vi "TestPFGVName.vi"() -> (0 "error out":errorcluster, 2 "Pass":bool)   [LabVIEW 2015]
uses:
  TypeDef/RoomsActionEnum.ctl
  TypeDef/PersonnelActions.ctl
  LVClasses/Flags/Flags.lvclass
  LVClasses/Room/Room.lvclass
panel:
  out "Read Name":string
  out "Write Name":string
  out "Read Personnel":string
  out "Read Personnel 2":string
  in  "PUID":string="d1"
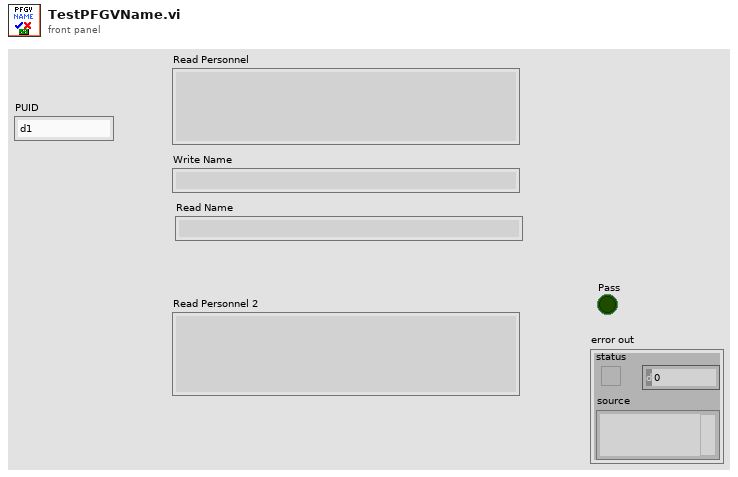
[diagram p1: front panel]
types:
  T1 = typedef "PersonnelActions.ctl" = enum16{"Init", "Read Personnel", "Add Personnel", "Remove Personnel", "Read Name", "Write Name", "Read Role", "Write Role", "Read PUID", "Write PUID", "Read Requests", "Add Requests", "Remove Requests"}
  T2 = typedef "RoomsActionEnum.ctl" = enum16{"Init", "Add Room", "Remove Room", "Read Room", "Read Flag", "Read Flag State", "Write Flag State", "Read Flag Color", "Write Flag Color", "Read Bed Vacant", "Write Bed Vacant", "Read Personnel", "Add Personnel", "Remove Personnel", "Read Requests", "Add Request", "Remove Request", "Read Beacon ID", "Write Beacon ID", "Write Bed URL", "Read Bed URL", "Read Rooms Numbers", "Write Flag"}
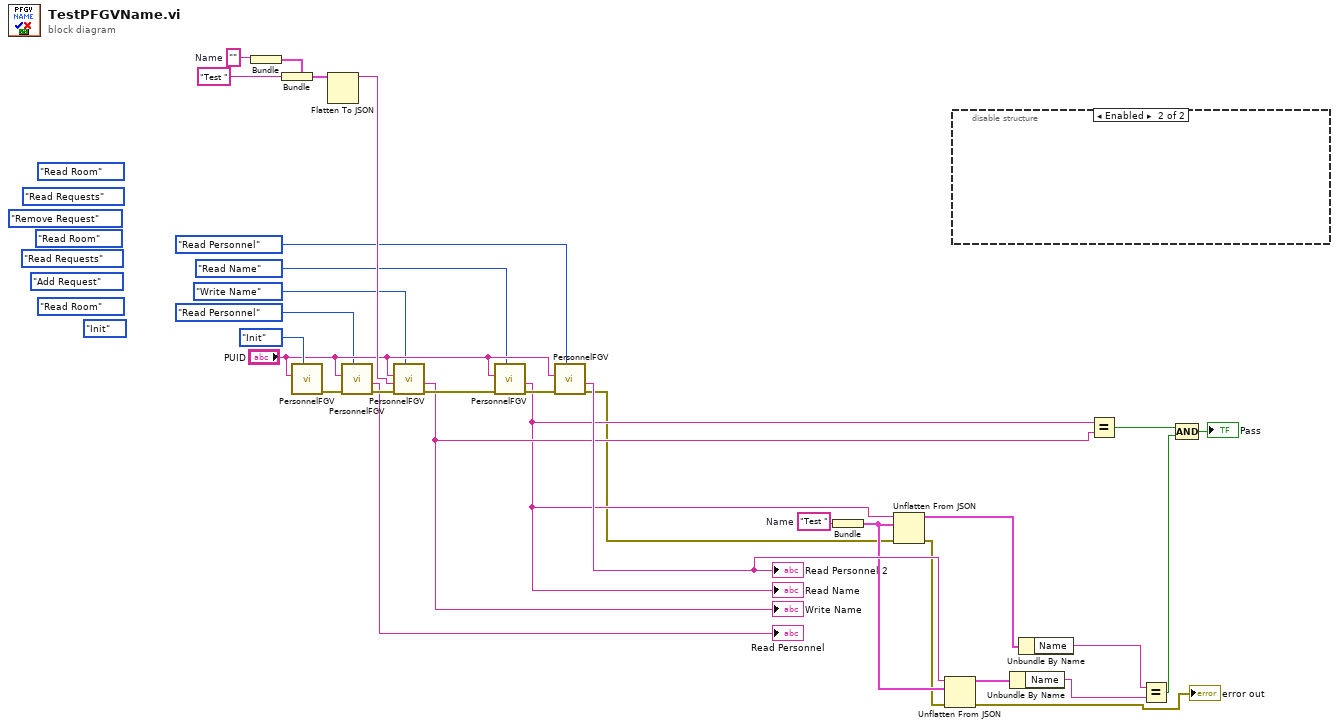
[diagram p0: block diagram]
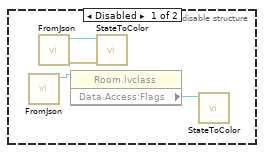
[diagram p2: hidden frame]
diagram:
  w11 = "Test "  # Name
  (unwired) RoomsActionEnum."Read Requests"
  (unwired) RoomsActionEnum."Remove Request"
  w27 = ""  # Name
  (unwired) RoomsActionEnum."Add Request"
  (unwired) RoomsActionEnum."Read Room"
  (unwired) RoomsActionEnum."Read Requests" ("Actions")
  (unwired) RoomsActionEnum."Read Room"
  (unwired) RoomsActionEnum."Read Room"
  (unwired) RoomsActionEnum."Init"
  n1 = Bundle("Name"=w27) -> (w26:cluster{"Name":string})  [unwired: 1 in]
  n2 = Bundle(cluster=w26, "Name"="Test " ("Request")) -> (w25:cluster{"Name":string})
  n3 = call "PersonnelFGV.vi"("Actions"=PersonnelActions."Init", "PUID"="PUID") -> ("error out"=w31:errorcluster)  [unwired: 8 in, 1 out]
  n4 = Flatten To JSON(anything=w25) -> (JSON string=w24:string)  [unwired: 2 in, 1 out]
  n5 = call "PersonnelFGV.vi"("Actions"=PersonnelActions."Read Personnel", "error in (no error)"=w31, "PUID"="PUID") -> ("error out"=w30:errorcluster, "Data Out"=→"Read Personnel":string)  [unwired: 7 in]
  n6 = call "PersonnelFGV.vi"("Actions"=PersonnelActions."Write Name", "error in (no error)"=w30, "Data In"=w24, "PUID"="PUID") -> ("error out"=w28:errorcluster, "Data Out"=w8:string)  [unwired: 6 in]
  "Write Name" <- w8
  n7 = call "PersonnelFGV.vi"("Actions"=PersonnelActions."Read Name", "error in (no error)"=w28, "PUID"="PUID") -> ("error out"=w29:errorcluster, "Data Out"=w7:string)  [unwired: 7 in]
  "Read Name" <- w7
  n8 = call "PersonnelFGV.vi"("Actions"=PersonnelActions."Read Personnel", "error in (no error)"=w29, "PUID"="PUID") -> ("error out"=w3:errorcluster, "Data Out"=w10:string)  [unwired: 7 in]
  "Read Personnel 2" <- w10
  n9 = Bundle("Name"=w11) -> (w4:cluster{"Name":string})  [unwired: 1 in]
  n10 = Unflatten From JSON(JSON string=w7, type and defaults=w4, error in (no error)=w3) -> (value=w6:cluster{"Name":string}, error out=w2:errorcluster)  [unwired: 4 in]
  n11 = Unflatten From JSON(JSON string=w10, type and defaults=w4, error in (no error)=w2) -> (value=w18:cluster{"Name":string}, error out=→"error out":errorcluster)  [unwired: 4 in]
  n12 = disable-structure shown="Enabled" {
    frame Disabled {
      n13 = call "FromJson.vi"() -> ("Room out"=w33:refnum<class "Room.lvclass">)  [unwired: 10 in, 1 out]
      n14 = call "FromJson.vi"() -> ("error out"=w35:errorcluster, "Flags out"=w34:refnum<class "Flags.lvclass">)  [unwired: 10 in]
      n15 = property class="Room.lvclass"(reference=w33) -> ("Data Access:Flags"=w32:refnum<class "Flags.lvclass">)  [unwired: 1 in, 2 out]
      n16 = call "StateToColor.vi"("error in (no error)"=w35, "Flags in"=w34) -> ()  [unwired: 7 in, 3 out]
      n17 = call "StateToColor.vi"("Flags in"=w32) -> ()  [unwired: 8 in, 3 out]
    }
    frame Enabled {
    }
  }
  n18 = Unbundle By Name(w18) -> ("Name"=w9:string)
  n19 = Unbundle By Name(w6) -> ("Name"=w5:string)
  n20 = Equal?(x=w7, y=w8) -> (x = y?=w22:bool)
  n21 = Equal?(x=w5, y=w9) -> (x = y?=w20:bool)
  n22 = Compound Arithmetic op=AND(w22, w20) -> (→"Pass":bool)
